vi "divide at end of cycle.vi"() -> ()   [LabVIEW 2010]
uses:
  <vilib>/rvi/FXPMathLib/FxpDiv/XNode/nifxpmath_Div.xnode
  <vilib>/rvi/FXPMathLib/FxpDiv/subVIs/nifxpmath_Div_SimConfig.ctl
  <vilib>/rvi/FXPMathLib/FxpDiv/simVIs/DllFxpDivTemp_sub.vi
panel:
  in  "ready for output (T)":bool=TRUE
  out "avg":i16
  out "output valid":bool
  in  "end of cycle":bool
  in  "divisor":u32
  out "sum out":i32
  in  "sum in":i32
  # "32 bit signed integer"
  # "32 bit unsigned integer"
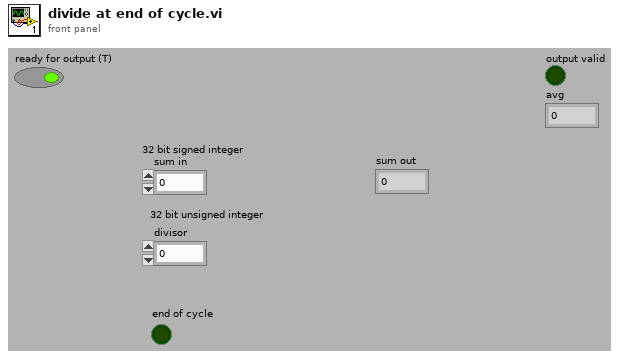
[diagram p1: front panel]
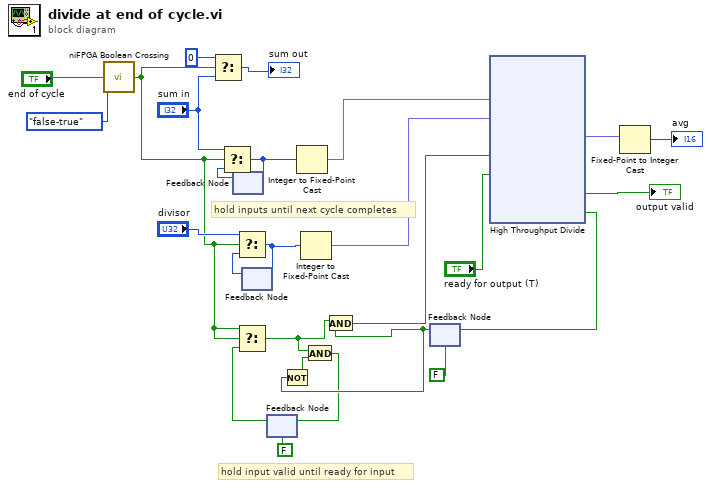
[diagram p0: block diagram]
diagram:
  # "hold input valid until ready for input"
  # "hold inputs until next cycle completes"
  n1 = call <vilib>:"niFPGA Boolean Crossing.vi"("input"="end of cycle", "direction"=enum8{"either", "false-true", "true-false"}."false-true") -> ("crossing"=w18:bool)  [unwired: 7 in]
  n2 = Select(t=0, s=w18, f="sum in") -> (s? t:f=→"sum out":i32)
  n3 = feedback #1() -> (w21:i32)  [unwired: 1 in]
  n4 = Select(t="sum in", s=w18, f=w21) -> (s? t:f=w7:i32)
  n5 = feedback-in #1(w7) -> ()
  n6 = feedback #2() -> (w19:u32)  [unwired: 1 in]
  n7 = Select(t="divisor", s=w18, f=w19) -> (s? t:f=w5:u32)
  n8 = feedback-in #2(w5) -> ()
  n9 = feedback #3(FALSE) -> (w10:bool)
  n10 = Select(t=w18, s=w18, f=w10) -> (s? t:f=w14:bool)
  n11 = Integer to Fixed-Point Cast(integer=w7) -> (fixed-point=w6:fxp<+/-,32,32>)  [unwired: 1 in]
  n12 = Integer to Fixed-Point Cast(integer=w5) -> (fixed-point=w4:fxp<+,32,32>)  [unwired: 1 in]
  n13 = feedback #4(FALSE ("ready for input")) -> (w13:bool)
  n14 = Not(x=w13) -> (.not. x?=w12:bool)
  n15 = And(x=w14, y=w12) -> (x .and. y?=w11:bool)
  n16 = feedback-in #3(w11) -> ()
  n17 = And(x=w14, y=w13) -> (x .and. y?=w15:bool)
  n18 = xnode "High Throughput Divide"("x"=w6, "y"=w4, "input valid"=w15, "ready for output (T)"="ready for output (T)") -> ("x/y"=w8:fxp<+/-,16,16>, "output valid"=→"output valid":bool, "ready for input"=w17:bool)
  n19 = feedback-in #4(w17) -> ()
  n20 = Fixed-Point to Integer Cast(1:w8) -> (0:→"avg":i16)
